vi "Registry Handle Master.vi"(6 "machine":string, 7 "action (get handles)":T2(ring)=enum."get handles", 8 "error in (no error)":errorcluster, 9 "remote key handle":u64 format="%.0x", 10 "key handle":u64 format="%.0x", 11 "refnum":T1) -> (0 "error out":errorcluster, 1 "remote key handle out":u64 format="%.0x", 2 "key handle out":u64 format="%.0x", 3 "refnum out":T1, 4 "machine out":string)   [LabVIEW 2020]
doc: "Manages a temporary repository for Registry key handles. Closes all key handles if calling VI becomes idle, if user aborts execution, for example.\n\nWarning: Incorrectly modifying the Registry can damage Windows and may even prevent you from starting Windows."
uses:
  Registry refnum.ctl
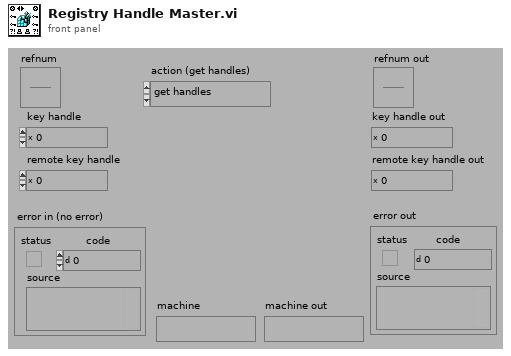
[diagram p1: front panel]
types:
  T1 = typedef "Registry refnum.ctl" = refnum<k1>
  T2 = enum16{"store handles", "dispose handles", "get handles"}
  T3 = cluster{"machine":string, "key handle":u64, "remote key handle":u64}
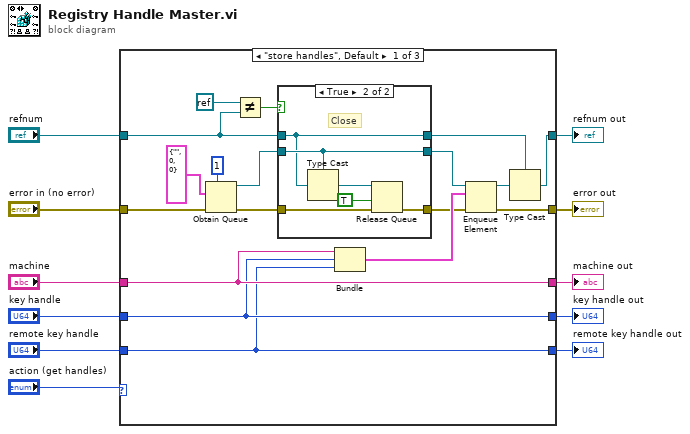
[diagram p0: block diagram]
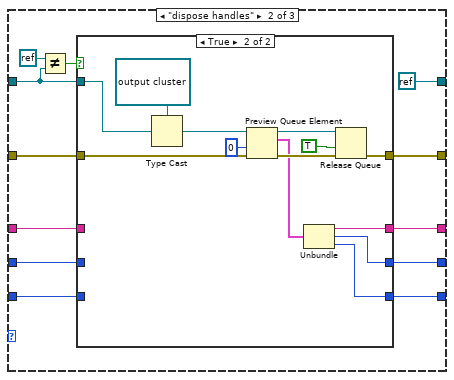
[diagram p3: hidden frame]
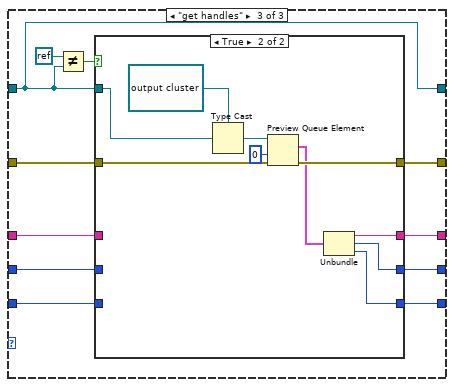
[diagram p5: hidden frame]
diagram:
  n1 = case shown="\"store handles\", Default" "action (get handles)" {
    tunnel: "refnum" -> [w13 w47 w72]
    tunnel: [w28 refnum<k0> refnum w72] -> w4
    tunnel: "error in (no error)" -> [w22 w50 w74]
    tunnel: "machine" -> [w17 w42 w70]
    tunnel: "key handle" -> [w16 w41 w69]
    tunnel: "remote key handle" -> [w15 w40 w68]
    tunnel: [w27 w49 w78] -> w5
    tunnel: [w17 w45 w77] -> w3
    tunnel: [w16 w44 w76] -> w2
    tunnel: [w15 w43 w75] -> w1
    frame "store handles", Default {
      n2 = Obtain Queue(max queue size (-1, unlimited)=1, element data type=T3 {"machine"="", "key handle"=0, "remote key handle"=0} ("output cluster"), error in (no error)=w22) -> (queue out=w21:refnum<queue>, error out=w19:errorcluster)  [unwired: 1 in, 2 out]
      n3 = Not Equal?(x=refnum<k0> refnum, y=w13) -> (x != y?=w12:bool)
      n4 = case shown="True" w12 {
        tunnel: w19 -> [w32 w36]
        tunnel: [w32 w37] -> w25
        tunnel: w13 -> [w30 w34]
        tunnel: w21 -> [w31 w35]
        tunnel: [w31 w35] -> w20
        tunnel: [w30 w34] -> w18
        frame False {
        }
        frame True {
          # "Close"
          n5 = Type Cast(type=w35, x=w34) -> (*(type *) &x=w38:refnum<queue>)
          n6 = Release Queue(queue=w38, force destroy? (F)=TRUE, error in (no error)=w36) -> (error out=w37:errorcluster)  [unwired: 2 out]
        }
      }
      n7 = Bundle("machine"=w17, "key handle"=w16, "remote key handle"=w15) -> (w26:T3)  [unwired: 1 out]
      n8 = Enqueue Element(queue=w20, element=w26, error in (no error)=w25) -> (queue out=w29:refnum<queue>, error out=w27:errorcluster)  [unwired: 2 out]
      n9 = Type Cast(type=w18, x=w29) -> (*(type *) &x=w28:T1)
    }
    frame "dispose handles" {
      n10 = Not Equal?(x=refnum<k0> refnum, y=w47) -> (x != y?=w46:bool)
      n11 = case shown="True" w46 {
        tunnel: w50 -> [w54 w60]
        tunnel: [w54 w67] -> w49
        tunnel: w47 -> [_ w66]
        tunnel: [w53 w57] -> w45
        tunnel: [w52 w56] -> w44
        tunnel: [w51 w55] -> w43
        tunnel: w42 -> [w53 _]
        tunnel: w41 -> [w52 _]
        tunnel: w40 -> [w51 _]
        frame False {
        }
        frame True {
          n12 = Type Cast(type=refnum<queue> refnum ("queue out"), x=w66) -> (*(type *) &x=w62:refnum<queue>)
          n13 = Preview Queue Element(queue=w62, timeout in ms (-1)=0, error in (no error)=w60) -> (queue out=w61:refnum<queue>, element=w58:T3, error out=w59:errorcluster)  [unwired: 1 out]
          n14 = Unbundle(w58) -> ("machine"=w57:string, "key handle"=w56:u64, "remote key handle"=w55:u64)
          n15 = Release Queue(queue=w61, force destroy? (F)=TRUE, error in (no error)=w59) -> (error out=w67:errorcluster)  [unwired: 2 out]
        }
      }
    }
    frame "get handles" {
      n16 = Not Equal?(x=refnum<k0> refnum, y=w72) -> (x != y?=w71:bool)
      n17 = case shown="True" w71 {
        tunnel: [w82 w91] -> w78
        tunnel: [w81 w89] -> w77
        tunnel: [w80 w88] -> w76
        tunnel: [w79 w87] -> w75
        tunnel: w74 -> [w82 w85]
        tunnel: w72 -> [_ w84]
        tunnel: w70 -> [w81 _]
        tunnel: w69 -> [w80 _]
        tunnel: w68 -> [w79 _]
        frame False {
        }
        frame True {
          n18 = Type Cast(type=refnum<queue> refnum ("queue out"), x=w84) -> (*(type *) &x=w92:refnum<queue>)
          n19 = Preview Queue Element(queue=w92, timeout in ms (-1)=0, error in (no error)=w85) -> (element=w90:T3, error out=w91:errorcluster)  [unwired: 2 out]
          n20 = Unbundle(w90) -> ("machine"=w89:string, "key handle"=w88:u64, "remote key handle"=w87:u64)
        }
      }
    }
  }
  "refnum out" <- w4
  "error out" <- w5
  "key handle out" <- w2
  "remote key handle out" <- w1
  "machine out" <- w3
